vi "DecipherRockPapScis.vi"(11 "A":string) -> (3 "Enum":T1(ring))   [LabVIEW 2021, in "2022.lvlib"]
uses:
  2022.lvlib
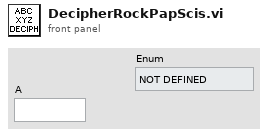
[diagram p1: front panel]
types:
  T1 = enum16{"NOT DEFINED", "Rock", "Paper", "Scissors"}
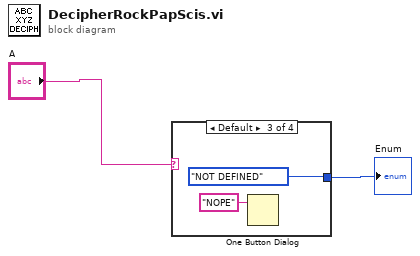
[diagram p0: block diagram]
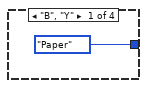
[diagram p2: hidden frame]
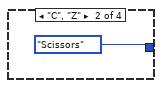
[diagram p3: hidden frame]
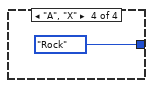
[diagram p4: hidden frame]
diagram:
  n1 = case shown="Default" "A" {
    tunnel: [T1."Paper" T1."Scissors" T1."NOT DEFINED" T1."Rock"] -> w1
    frame "B", "Y" {
    }
    frame "C", "Z" {
    }
    frame Default {
      n2 = One Button Dialog(message="NOPE") -> ()  [unwired: 1 in, 1 out]
    }
    frame "A", "X" {
    }
  }
  "Enum" <- w1
